vi "Test.vi"() -> ()   [LabVIEW 2020]
panel:
  out "appended path":path
  out "path":path
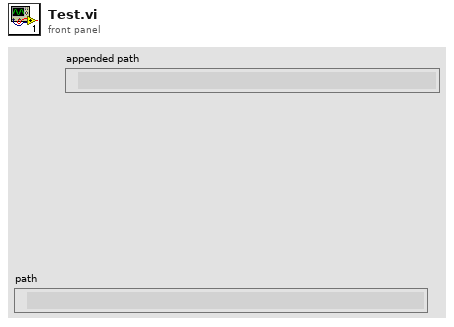
[diagram p1: front panel]
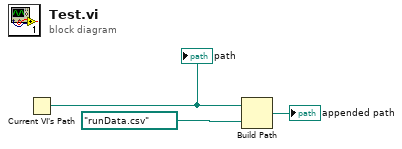
[diagram p0: block diagram]
diagram:
  n1 = Current VI's Path() -> (path=w1:path)
  "path" <- w1
  n2 = Build Path(base path=w1, name or relative path=path "runData.csv") -> (appended path=→"appended path":path)
